vi "Voltmeter error correction.vi"(4 "Относителоьная погрешность определения Rвн, %":dbl, 5 "Rвх вольтметра , Ом":dbl, 6 "Rвн источинка, Ом":dbl, 7 "Показания вольтметра , В":dbl) -> (0 "Неисключенная методическая погрешность , В":dbl, 1 "Исправленные показания , В":dbl, 2 "Поправка , В":dbl, 3 "Методичкая погрешность , В":dbl)   [LabVIEW 2013]
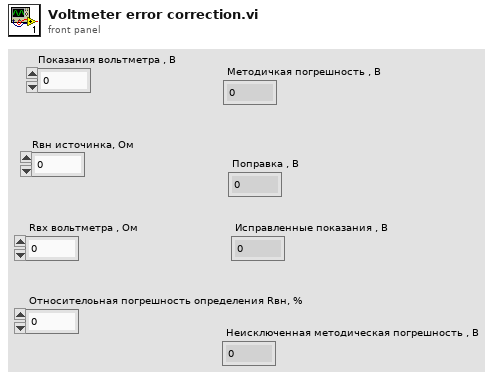
[diagram p1: front panel]
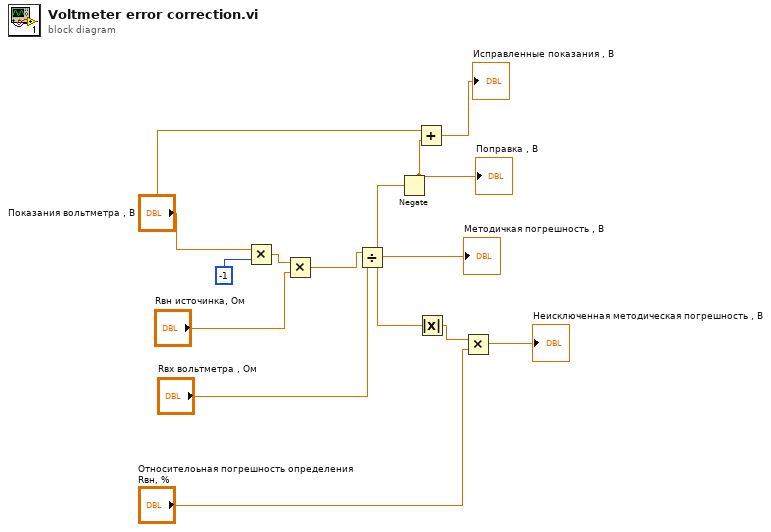
[diagram p0: block diagram]
diagram:
  n1 = Multiply(x="Показания вольтметра , В", y=-1) -> (x*y=w11:dbl)
  n2 = Multiply(x=w11, y="Rвн источинка, Ом") -> (x*y=w9:dbl)
  n3 = Divide(x=w9, y="Rвх вольтметра , Ом") -> (x/y=w4:dbl)
  "Методичкая погрешность , В" <- w4
  n4 = Negate(x=w4) -> (-x=w2:dbl)
  "Поправка , В" <- w2
  n5 = Add(x="Показания вольтметра , В", y=w2) -> (x+y=→"Исправленные показания , В":dbl)
  n6 = Absolute Value(x=w4) -> (abs(x)=w7:dbl)
  n7 = Multiply(x=w7, y="Относителоьная погрешность определения Rвн, %") -> (x*y=→"Неисключенная методическая погрешность , В":dbl)
